vi "Scale_Noise_floor_to_Volts.vi"(7 "1":T1={"Cal_"={"Fine"=0.000213623046875, "Coarse_"=4194303.0}, "Beac"={"Fine"=0.000213623046875, "Coarse_"=4194303.0}, "Scale"={"Step4"=0.0, "Step5"=4194303.0, "Step6"=1.0, "Step7"=10000.0}, "Offset"=0.0, "Scale_Noise"=4194303.0, "Scale_Step1"=65535.0, "Scale_In_RT"=1.0, "ScaleMeas"=0.999969482421875, "FreqsToRemove"=[0, 1633], "Width"=[0, 1633], "ScaleMeasEnum"=enum."50", "FilterEnab"=enum."Step 1"}, 11 "spectrum in":dbl[](array[numeric])) -> (3 "Volts":dbl[](array[numeric]))   [LabVIEW 2018]
uses:
  Controls/Clusts/FP_UserTargetConfig.ctl
  Controls/Clusts/FreqShift.ctl
  Controls/Clusts/FPGA_Scale.ctl
  Controls/Enums/ScaleMeasure.ctl
  Controls/RadioButtons/FilterEnableRadio.ctl
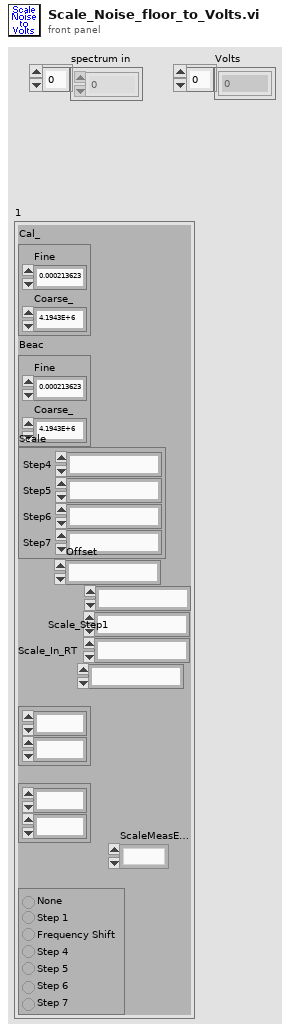
[diagram p1: front panel]
types:
  T1 = typedef "FP_UserTargetConfig.ctl" = cluster{"Cal_":T2, "Beac":T2, "Scale":T3, "Offset":fxp<+/-,16,16>, "Scale_Noise":fxp<+/-,30,30>, "Scale_Step1":fxp<+/-,17,17>, "Scale_In_RT":ext, "ScaleMeas":fxp<+/-,16,1>, "FreqsToRemove":i32[], "Width":i32[], "ScaleMeasEnum":T4, "FilterEnab":T5}
  T2 = typedef "FreqShift.ctl" = cluster{"Fine":dbl, "Coarse_":dbl}
  T3 = typedef "FPGA_Scale.ctl" = cluster{"Step4":fxp<+/-,23,23>, "Step5":fxp<+/-,23,23>, "Step6":fxp<+/-,23,23>, "Step7":fxp<+/-,23,23>}
  T4 = typedef "ScaleMeasure.ctl" = enum16{"1", "10", "50", "42"}
  T5 = typedef "FilterEnableRadio.ctl" = enum32{"None", "Step 1", "Frequency Shift", "Step 4", "Step 5", "Step 6", "Step 7"}
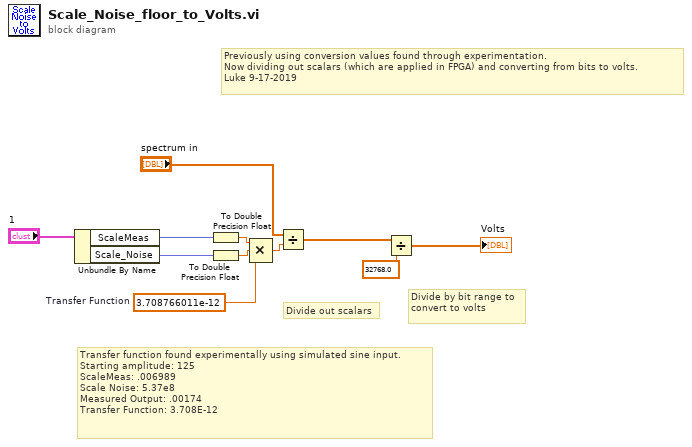
[diagram p0: block diagram]
diagram:
  w1 = 3.708766011e-12  # Transfer Function
  # "Transfer function found experimentally using simulated sine input.\nStarting amplitude: 125\nScaleMeas: .006989\nScale Noise: 5.37e8\nMeasured Output: .00174\nTransfer Function: 3.708E-12"
  # "Divide out scalars"
  # "Divide by bit range to convert to volts"
  # "Previously using conversion values found through experimentation. \nNow dividing out scalars (which are applied in FPGA) and converting from bits to volts.\nLuke 9-17-2019"
  n1 = Unbundle By Name("1") -> ("ScaleMeas"=w10:fxp<+/-,16,1>, "Scale_Noise"=w9:fxp<+/-,30,30>)
  n2 = To Double Precision Float(number=w10) -> (double precision float=w8:dbl)
  n3 = To Double Precision Float(number=w9) -> (double precision float=w7:dbl)
  n4 = Compound Arithmetic op=MULTIPLY(w8, w7, w1) -> (w6:dbl)
  n5 = Divide(x="spectrum in", y=w6) -> (x/y=w5:dbl[])
  n6 = Divide(x=w5, y=32768.0) -> (x/y=→"Volts":dbl[])
